vi "createStreamReader.vi"(4 "Read Timeout Type (Any)":T1 items=["daqReadTimeoutTypeAny", "daqReadTimeoutTypeAll"], 6 "Read Mode (raw value)":T2=2 items=["daqReadModeUnscaled", "daqReadModeScaled", "daqReadModeRawValue"], 7 "Domain Type (Int64)":T3=10 items=["daqSampleTypeInvalid", "daqSampleTypeFloat32", "daqSampleTypeFloat64", "daqSampleTypeUInt8", "daqSampleTypeInt8", "daqSampleTypeUInt16", "daqSampleTypeInt16", "daqSampleTypeUInt32", "daqSampleTypeInt32", "daqSampleTypeUInt64", "daqSampleTypeInt64", "daqSampleTypeRangeInt64", "daqSampleTypeComplexFloat32", "daqSampleTypeComplexFloat64", "daqSampleTypeBinary", "daqSampleTypeString", "daqSampleTypeStruct", "daqSampleTypeNull", "daqSampleType_count"], 8 "error in (no error)":errorcluster, 9 "Sample Type (Float64)":T3=2 items=["daqSampleTypeInvalid", "daqSampleTypeFloat32", "daqSampleTypeFloat64", "daqSampleTypeUInt8", "daqSampleTypeInt8", "daqSampleTypeUInt16", "daqSampleTypeInt16", "daqSampleTypeUInt32", "daqSampleTypeInt32", "daqSampleTypeUInt64", "daqSampleTypeInt64", "daqSampleTypeRangeInt64", "daqSampleTypeComplexFloat32", "daqSampleTypeComplexFloat64", "daqSampleTypeBinary", "daqSampleTypeString", "daqSampleTypeStruct", "daqSampleTypeNull", "daqSampleType_count"], 10 "connectedSignal":refnum<class "ISignal.lvclass">, 11 "IStreamReader in":refnum<class "IStreamReader.lvclass">) -> (0 "error out":errorcluster, 3 "IStreamReader out":refnum<class "IStreamReader.lvclass">)   [LabVIEW 2022 SP3, in "openDAQ.lvlib" / "IBaseObject.lvlib" / "IReader.lvlib" / "ISampleReader.lvlib" / "IStreamReader.lvlib" / "IStreamReader.lvclass"]
uses:
  <instrlib>/openDAQ/Public/Classes/IBaseObject/IBaseObject.lvclass/IBaseObject.ctl
  <instrlib>/openDAQ/Public/Classes/IBaseObject/Accessor/Read reference.vi
  <instrlib>/openDAQ/Public/Classes/IBaseObject/Accessor/Write reference.vi
  <instrlib>/openDAQ/Public/Classes/IStreamReader/IStreamReader.lvclass
  <instrlib>/openDAQ/Public/Classes/IStreamReader/IStreamReader.lvclass/IStreamReader.ctl
  <instrlib>/openDAQ/Binaries/Windows/x86/copendaq32.dll
  <instrlib>/openDAQ/Public/Classes/ISignal/ISignal.lvclass
  <instrlib>/openDAQ/Public/TypeDef/daqSampleType.ctl
  <instrlib>/openDAQ/openDAQ.lvlib
  <instrlib>/openDAQ/Public/TypeDef/daqReadMode.ctl
  <instrlib>/openDAQ/Public/TypeDef/daqReadTimeoutType.ctl
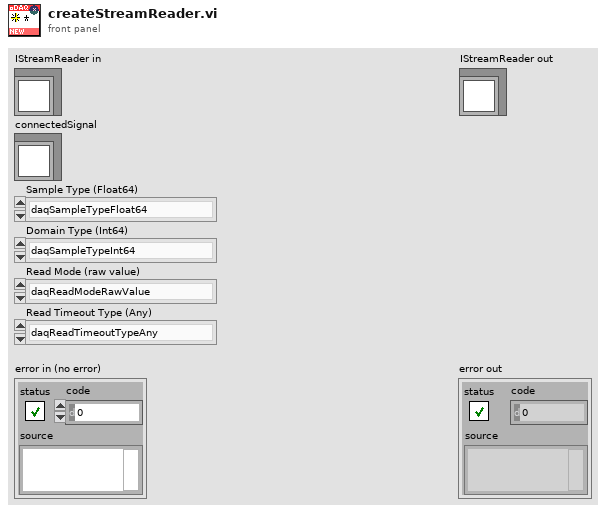
[diagram p1: front panel]
types:
  T1 = typedef "openDAQ.lvlib/daqReadTimeoutType.ctl" = u16
  T2 = typedef "openDAQ.lvlib/daqReadMode.ctl" = u16
  T3 = typedef "openDAQ.lvlib/daqSampleType.ctl" = u16
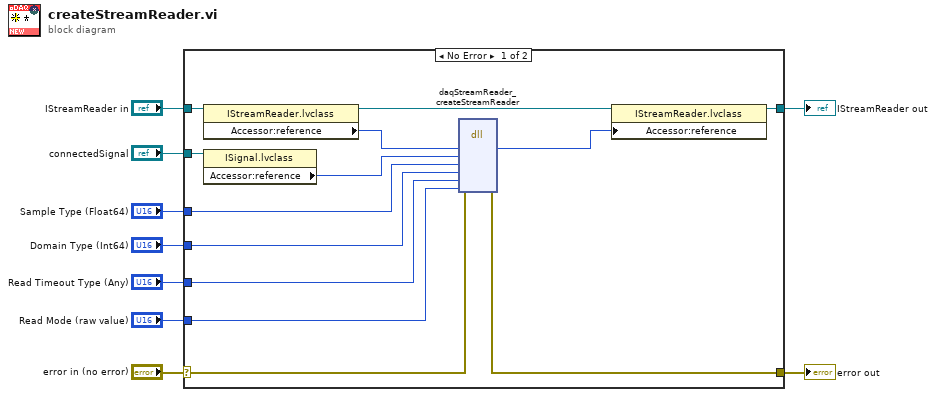
[diagram p0: block diagram]
diagram:
  n1 = case shown="No Error" "error in (no error)" {
    selector: "error in (no error)" -> [w22 w24]
    tunnel: [w21 w24] -> w8
    tunnel: [w17 w23] -> w6
    tunnel: "IStreamReader in" -> [w20 w23]
    tunnel: "connectedSignal" -> [w15 _]
    tunnel: "Sample Type (Float64)" -> [w13 _]
    tunnel: "Domain Type (Int64)" -> [w12 _]
    tunnel: "Read Timeout Type (Any)" -> [w11 _]
    tunnel: "Read Mode (raw value)" -> [w10 _]
    frame No Error {
      n2 = property class="IStreamReader.lvclass"(reference=w20) -> (reference out=w18:refnum<class "IStreamReader.lvclass">, "Accessor:reference"=w19:i64)  [unwired: 1 in, 1 out]
      n3 = property class="ISignal.lvclass"(reference=w15) -> ("Accessor:reference"=w14:i64)  [unwired: 1 in, 2 out]
      n4 = dll-call lib="C:/Program Files (x86)/National Instruments/LabVIEW 2022/instr.lib/openDAQ/Binaries/Windows/x86/copendaq*.*" fn="daqStreamReader_createStreamReader"(error in=w22, "reader"=w19, "connectedSignal"=w14, "sampleType"=w13, "domainType"=w12, "readMode"=w11, "timeout"=w10) -> (error out=w21:errorcluster, "reader"=w16:i64)  [unwired: 8 in, 1 out]
      n5 = property class="IStreamReader.lvclass"(reference=w18, "Accessor:reference"=w16) -> (reference out=w17:refnum<class "IStreamReader.lvclass">)  [unwired: 1 in, 1 out]
    }
    frame Error {
    }
  }
  "error out" <- w8
  "IStreamReader out" <- w6
